vi "Lift Close.vi"(1 "error in (no error)":errorcluster) -> (0 "error out":errorcluster)   [LabVIEW 2014]
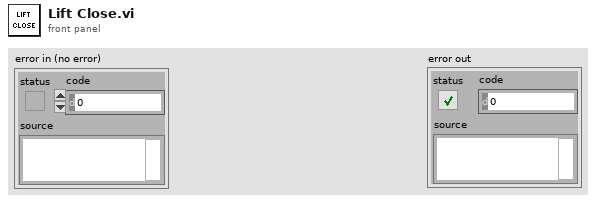
[diagram p1: front panel]
types:
  T1 = typedef "WPI_MotorControlDeviceRef.ctl" = cluster{"DeviceStatus":errorcluster, "Type":T2, "PWM":cluster{"Controller":T3, "PWM Channel":T4, "DeadBand":T5}, "CAN":cluster{"Device Number":u8, "Control Mode":T6, "Semaphore":T7, "Max Vout":dbl, "TalonSRX Control Mode":T8}, "Invert":bool, "TransformRef":T9, "InvTransformRef":T9}
  T2 = typedef "WPI_MotorControlType.ctl" = enum16{"PWM", "CAN", "CANTalonSRX"}
  T3 = typedef "FPGA_TypedefDigitalModule.ctl" = enum16{"Controller 1"}
  T4 = typedef "FPGA_DIOPWMChannel.ctl" = enum8{"PWM 0", "PWM 1", "PWM 2", "PWM 3", "PWM 4", "PWM 5", "PWM 6", "PWM 7", "PWM 8", "PWM 9", "PWM MXP 0", "PWM MXP 1", "PWM MXP 2", "PWM MXP 3", "PWM MXP 4", "PWM MXP 5", "PWM MXP 6", "PWM MXP 7", "PWM MXP 8", "PWM MXP 9", "Invalid"}
  T5 = typedef "WPI_PWMDeadband.ctl" = cluster{"Name":string, "maxPositivePwm":i32, "minPositivePwm":i32, "centerPwm":i32, "maxNegativePwm":i32, "minNegativePwm":i32, "angularRange":u16}
  T6 = typedef "WPI_CANJaguar_ControlMode.ctl" = enum8{"Percent VBus", "Current", "Speed", "Position", "Voltage"}
  T7 = typedef "Semaphore RefNum" = refnum<k1>
  T8 = typedef "WPI_CANTalonSRX_APIControlMode.ctl" = enum8{"Percent VBus", "Speed", "Position", "Slave", "Unchanged / Invalid"}
  T9 = typedef "WPI_PWMTransform_ConPane.ctl" = refnum<vi>
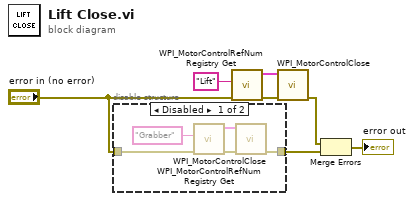
[diagram p0: block diagram]
diagram:
  n1 = disable-structure shown="Disabled" {
    disable-tunnel: "error in (no error)" -> [w9 _]
    disable-tunnel: [w8 _] -> w2
    frame Disabled {
      n2 = call <vilib>:"WPI_MotorControlRefNum Registry Get.vi"("error in (no error)"=w9, "refnum name"="Grabber") -> ("error out"=w11:errorcluster, "MotorControlDevRef"=w12:T1)  [unwired: 8 in]
      n3 = call <vilib>:"WPI_MotorControlClose.vi"("error in (no error)"=w11, "MotorControlDevRef"=w12) -> ("error out"=w8:errorcluster)  [unwired: 9 in]
    }
    frame Enabled {
    }
  }
  n4 = call <vilib>:"WPI_MotorControlRefNum Registry Get.vi"("error in (no error)"="error in (no error)", "refnum name"="Lift") -> ("error out"=w5:errorcluster, "MotorControlDevRef"=w7:T1)  [unwired: 8 in]
  n5 = call <vilib>:"WPI_MotorControlClose.vi"("error in (no error)"=w5, "MotorControlDevRef"=w7) -> ("error out"=w3:errorcluster)  [unwired: 9 in]
  n6 = Merge Errors(w3, w2) -> (→"error out":errorcluster)
